vi "General-GetGaussianArray.vi"(0 "tiempo (ms)":dbl, 1 "Amplitud":dbl, 2 "t0 (ms)":dbl, 3 "Sigma (ms)":dbl, 4 "#samples":u32) -> (5 "Y out":dbl[](array[numeric]), 6 "t out":sgl[](array[numeric]))   [LabVIEW 2010]
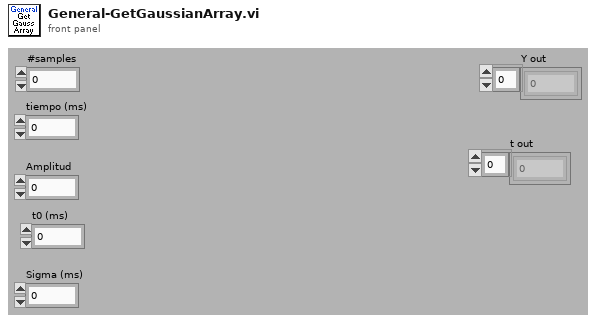
[diagram p1: front panel]
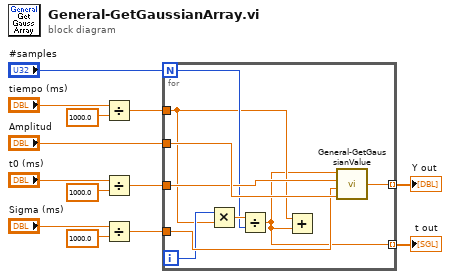
[diagram p0: block diagram]
diagram:
  n1 = Divide(x="tiempo (ms)", y=sgl 1000.0) -> (x/y=w1:dbl)
  n2 = Divide(x="t0 (ms)", y=sgl 1000.0) -> (x/y=w9:dbl)
  n3 = Divide(x="Sigma (ms)", y=sgl 1000.0) -> (x/y=w10:dbl)
  n4 = for {
    N: "#samples" -> [w18]
    tunnel: [w14] -> w11 mode=indexing
    tunnel: "Amplitud" -> [w21]
    tunnel: w10 -> [w20]
    tunnel: w9 -> [w19]
    tunnel: w1 -> [w16]
    tunnel: [w15] -> w13 mode=indexing
    i -> [w17]
    n5 = Multiply(x=w17, y=w16) -> (x*y=w22:dbl)
    n6 = Divide(x=w22, y=w18) -> (x/y=w15:dbl)
    n7 = Add(x=w16, y=w15) -> ()  [unwired: 1 out]
    n8 = call "General-GetGaussianValue.vi"("Amplitud"=w21, "sigma"=w20, "miu"=w19, "x"=w15) -> ("out"=w14:dbl)
  }
  "t out" <- w13
  "Y out" <- w11
